vi "DFD Butterworth Order Estimation.vi"(6 "fs [Hz]":dbl=1.0 format="%.2f", 7 "filter type":T3(ring), 8 "error in (no error)":errorcluster, 10 "ripple specs":T1={"passband"=0.1, "stopband"=60.0, "dB/linear? (T: dB)"=TRUE}, 11 "freq specs [Hz]":T2={"fpass 1"=0.2, "fstop 1"=0.3, "fpass 2 "=0.0, "fstop 2"=0.0}) -> (0 "error out":errorcluster, 1 "low cutoff freq [Hz]":dbl, 2 "high cutoff freq [Hz]":dbl, 3 "estimated order":i32)   [LabVIEW 2017, in "NI_DigFilterLicensed.lvlib"]
doc: "Estimates the Butterworth filter order."
uses:
  <vilib>/addons/Digital Filter Design/NI_DigFilterLicensed.lvlib
  <vilib>/addons/Digital Filter Design/_Objects.llb/DFD Filter Frequence Specification (Design).ctl
  <vilib>/addons/Digital Filter Design/_Objects.llb/DFD Filter Ripple Specification (Design).ctl
  <vilib>/addons/Digital Filter Design/NI_DigFilter_Design.lvlib
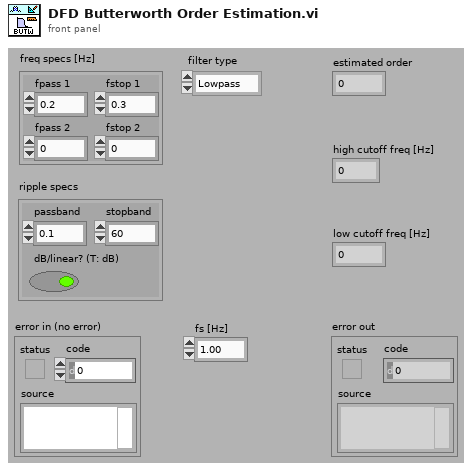
[diagram p1: front panel]
types:
  T1 = typedef "NI_DigFilterLicensed.lvlib/DFD Filter Ripple Specification (Design).ctl" = cluster{"passband":dbl, "stopband":dbl, "dB/linear? (T: dB)":bool}
  T2 = typedef "NI_DigFilterLicensed.lvlib/DFD Filter Frequence Specification (Design).ctl" = cluster{"fpass 1":dbl, "fstop 1":dbl, "fpass 2 ":dbl, "fstop 2":dbl}
  T3 = enum16{"Lowpass", "Highpass", "Bandpass", "Bandstop"}
  T4 = enum16{"Butterworth", "Chebyshev", "Inverse Chebyshev", "Elliptic", "Bessel"}
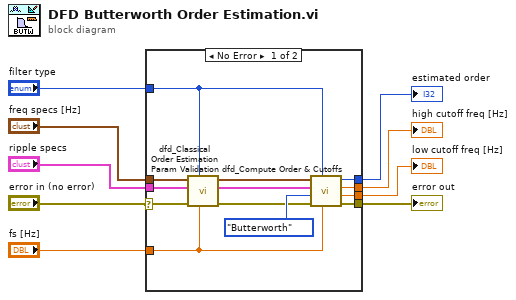
[diagram p0: block diagram]
diagram:
  n1 = case shown="No Error" "error in (no error)" {
    selector: "error in (no error)" -> [w10 w23]
    tunnel: [w22 _] -> w9
    tunnel: "fs [Hz]" -> [w21 _]
    tunnel: "filter type" -> [w20 _]
    tunnel: "freq specs [Hz]" -> [w19 _]
    tunnel: [w14 _] -> w5
    tunnel: [w13 _] -> w4
    tunnel: [w12 w23] -> w3
    tunnel: "ripple specs" -> [w11 _]
    frame No Error {
      n2 = call <vilib>:"dfd_Classical Order Estimation Param Validation.vi"("fs [Hz]"=w21, "filter type"=w20, "error in (no error)"=w10, "ripple specs"=w11, "freq specs [Hz]"=w19) -> ("error out"=w17:errorcluster, "dup ripple specs"=w15:T1, "dup freq specs [Hz]"=w16:T2)  [unwired: 1 in, 3 out]
      n3 = call <vilib>:"dfd_Compute Order & Cutoffs.vi"("fs [Hz]"=w21, "filter type"=w20, "error in (no error)"=w17, "design method"=T4."Butterworth", "ripple specs"=w15, "freq specs [Hz]"=w16) -> ("error out"=w12:errorcluster, "low cutoff freq: fl"=w13:dbl, "high cutoff freq: fh"=w14:dbl, "N"=w22:i32)  [unwired: 2 out]
    }
    frame Error {
    }
  }
  "estimated order" <- w9
  "error out" <- w3
  "high cutoff freq [Hz]" <- w5
  "low cutoff freq [Hz]" <- w4
